vi "calculate #seqs.vi"(8 "error in (no error)":errorcluster, 11 "S4ICS in":refnum<class "S4ICS.lvclass">) -> (0 "error out":errorcluster, 2 "#seqs":i16, 3 "S4ICS out":refnum<class "S4ICS.lvclass">)   [LabVIEW 2018]
uses:
  S4ICS.lvclass
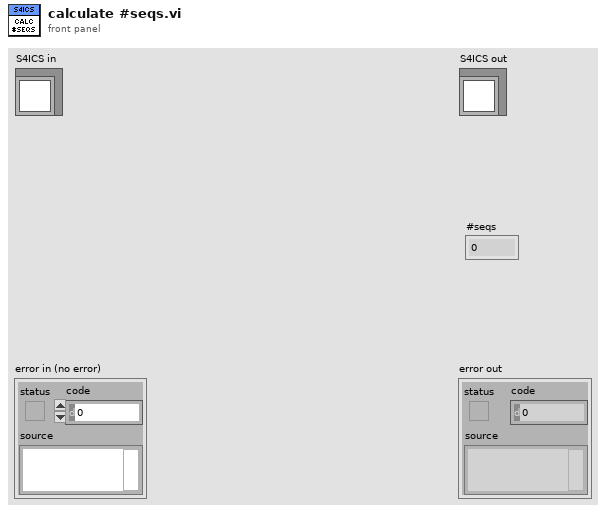
[diagram p1: front panel]
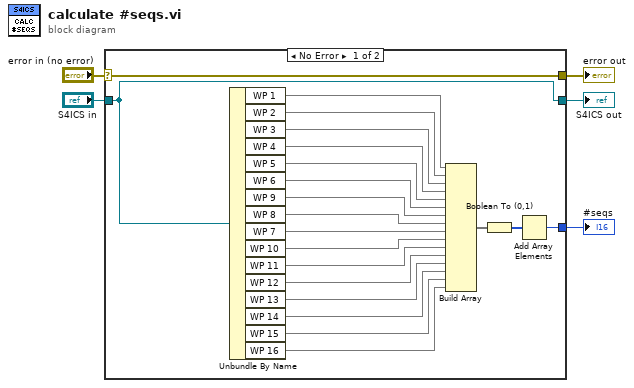
[diagram p0: block diagram]
diagram:
  n1 = case shown="No Error" "error in (no error)" {
    selector: "error in (no error)" -> [w26 w28]
    tunnel: [w26 w28] -> w4
    tunnel: [w9 w27] -> w2
    tunnel: "S4ICS in" -> [w9 w27]
    tunnel: [w6 _] -> w1
    frame No Error {
      n2 = Unbundle By Name(w9) -> ("WP 1"=w25, "WP 2"=w24, "WP 3"=w23, "WP 4"=w22, "WP 5"=w21, "WP 6"=w20, "WP 9"=w19, "WP 8"=w18, "WP 7"=w17, "WP 10"=w16, "WP 11"=w15, "WP 12"=w14, "WP 13"=w13, "WP 14"=w12, "WP 15"=w11, "WP 16"=w10)
      n3 = Build Array(w25, w24, w23, w22, w21, w20, w19, w18, w17, w16, w15, w14, w13, w12, w11, w10) -> (w8:void[])
      n4 = Boolean To (0,1)(Boolean=w8) -> (0, 1=w7:i16[])
      n5 = Add Array Elements(numeric array=w7) -> (sum=w6:i16)
    }
    frame Error {
    }
  }
  "error out" <- w4
  "S4ICS out" <- w2
  "#seqs" <- w1
